vi "Configure Event Search (Serial Bus - M1553).vi"(7 "Data Pattern (00000000000)":string="00000000000", 8 "error in (no error)":errorcluster, 9 "Remote Terminal Address (0)":i32, 10 "Search Operation (1: Command Start)":i32(ring)=1 items=["Data Start", "Command Start", "RTA", "RTA11", "Parity Error", "Sync Error", "Manchester Encoding Error"], 11 "VISA resource name":refnum<visa-resource-name>) -> (0 "error out":errorcluster, 3 "VISA resource name out":refnum<visa-resource-name>)   [LabVIEW 2010, in "Agilent 2000 3000 X-Series.lvlib"]
doc: "Configures the event search of MIL- STD- 1553 bus."
uses:
  <instrlib>/Agilent 2000 3000 X-Series/Agilent 2000 3000 X-Series.lvlib
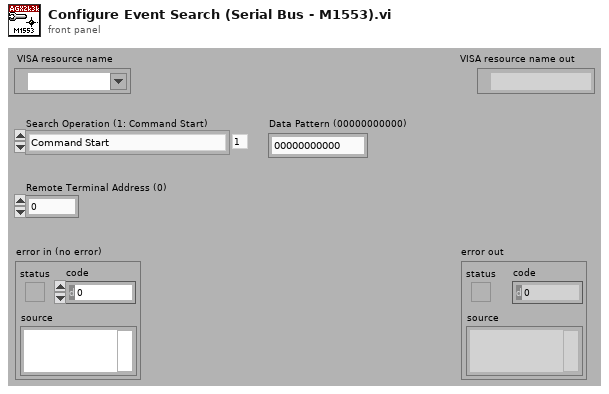
[diagram p1: front panel]
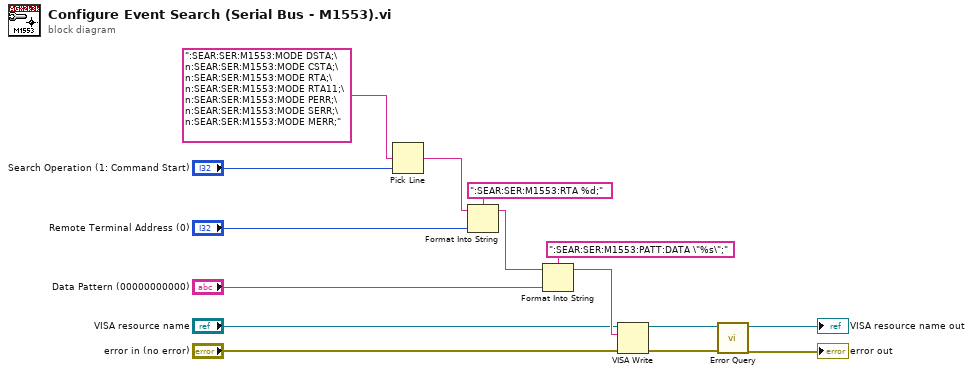
[diagram p0: block diagram]
diagram:
  n1 = Pick Line(multi-line string=":SEAR:SER:M1553:MODE DSTA;\n:SEAR:SER:M1553:MODE CSTA;\n:SEAR:SER:M1553:MODE RTA;\n:SEAR:SER:M1553:MODE RTA11;\n:SEAR:SER:M1553:MODE PERR;\n:SEAR:SER:M1553:MODE SERR;\n:SEAR:SER:M1553:MODE MERR;", line index="Search Operation (1: Command Start)") -> (output string=w13:string)  [unwired: 1 out]
  n2 = Format Into String(format string=":SEAR:SER:M1553:RTA %d;", initial string=w13, "Remote Terminal Address (0)") -> (resulting string=w10:string)  [unwired: 1 in, 1 out]
  n3 = Format Into String(format string=":SEAR:SER:M1553:PATT:DATA \"%s\";", initial string=w10, "Data Pattern (00000000000)") -> (resulting string=w7:string)  [unwired: 1 in, 1 out]
  n4 = VISA Write(VISA resource name="VISA resource name", write buffer=w7, error in (no error)="error in (no error)") -> (VISA resource name out=w4:refnum<visa-resource-name>, error out=w3:errorcluster)  [unwired: 1 out]
  n5 = call <instrlib>:"Error Query.vi"("error in (no error)"=w3, "VISA resource name"=w4) -> ("error out"=→"error out":errorcluster, "VISA resource name out"=→"VISA resource name out":refnum<visa-resource-name>)  [unwired: 8 out]
